vi "Write to File.vi"(8 "error in":errorcluster, 10 "File Actor In":refnum<class "File Actor.lvclass">, 11 "Exe Write Main in":refnum<class "Exe Write Main.lvclass">) -> (0 "error out":errorcluster, 2 "File Actor Out":refnum<class "File Actor.lvclass">)   [LabVIEW 2014, in "Controller.lvlib" / "Exe Write Main.lvclass"]
doc: "In this command, we pole the MAP DVR which contains all of the data that is to be written to file...."
uses:
  Exe Write Main.lvclass
  File Actor/File Actor.lvclass
  File Actor/File Actor.lvclass/File Actor.ctl
  SuperActor/Ex Nested.lvclass/Ex Nested.ctl
  Exe Write Main.lvclass/Exe Write Main.ctl
  reusable/Data/Data.lvclass
  File Actor/Read Save DVR.vi
  File Actor/Read File DVR.vi
  SuperActor/Read Log Session.vi
  <userlib>/_Session Fwk/Session - Root.lvclass
  reusable/Session APIs/Session Log/System Log.lvclass
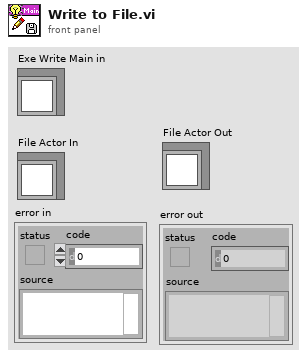
[diagram p1: front panel]
types:
  T1 = typedef "Session - Root.lvclass/Session Handle.ctl" = refnum<data-value>
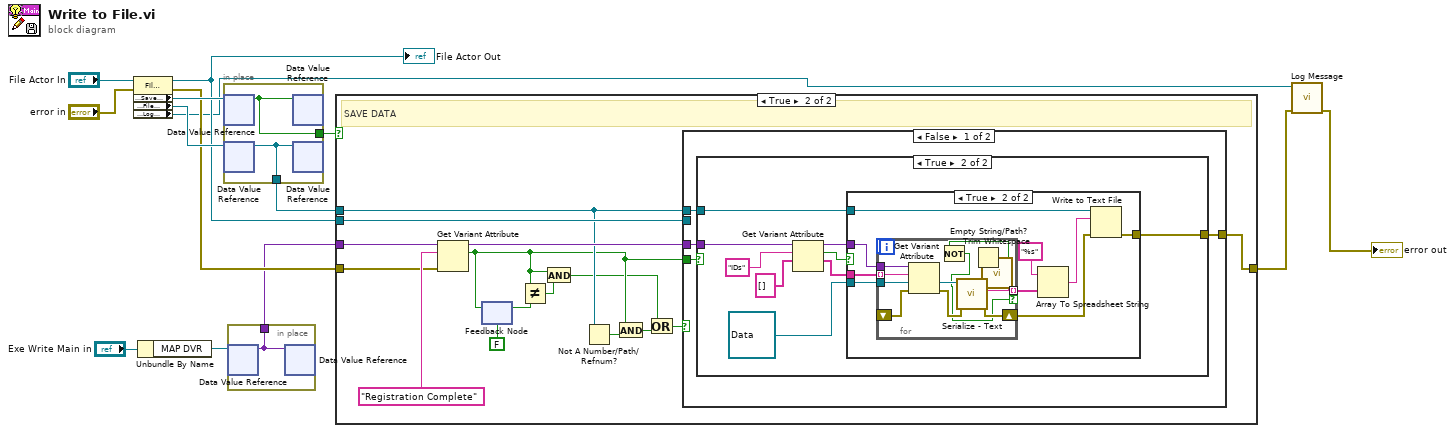
[diagram p0: block diagram]
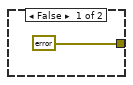
[diagram p4: hidden frame]
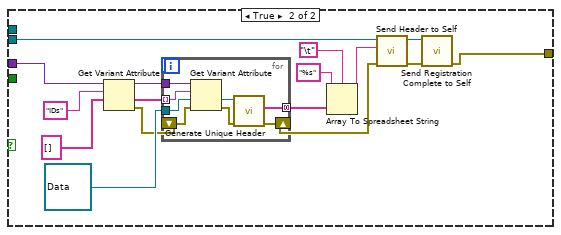
[diagram p5: hidden frame]
diagram:
  n1 = property class="File Actor"(reference="File Actor In", error in="error in") -> (reference out=w4:refnum<class "File Actor.lvclass">, error out=w8:errorcluster, "Accessors:Save DVR"=w13:refnum<data-value>, "Accessors:File DVR"=w11:refnum<data-value>, "Accessors:Log Session"=w3:T1)
  "File Actor Out" <- w4
  n2 = Unbundle By Name("Exe Write Main in") -> ("MAP DVR"=w6:refnum<data-value>)
  n3 = in-place {
    in-place-border: [w16] -> w12
    in-place-border: [w15] -> w10
    n4 = in-place-dvr #1(w13) -> (w16:bool)  [unwired: 1 out]
    n5 = in-place-dvr #2(w11) -> (w15:refnum<file>)  [unwired: 1 out]
    n6 = in-place-dvr #1(w16) -> ()  [unwired: 2 out]
    n7 = in-place-dvr #2(w15) -> ()  [unwired: 2 out]
  }
  n8 = in-place {
    in-place-border: [w17] -> w5
    n9 = in-place-dvr #3(w6) -> (w17:variant)  [unwired: 1 out]
    n10 = in-place-dvr #3(w17) -> ()  [unwired: 2 out]
  }
  n11 = case shown="True" w12 {
    tunnel: [w18 w33] -> w2
    tunnel: w10 -> [_ w24]
    tunnel: w8 -> [w18 w25]
    tunnel: w5 -> [_ w32]
    tunnel: w4 -> [_ w27]
    frame False {
      # "NO SAVE"
    }
    frame True {
      # "SAVE DATA"
      n12 = Get Variant Attribute(Variant=w32, name="Registration Complete", error in=w25) -> (duplicate Variant=w30:variant, found=w22:bool)  [unwired: 1 in, 2 out]
      n13 = feedback-in #4(w22) -> ()
      n14 = feedback #4(FALSE) -> (w29:bool)
      n15 = Not Equal?(x=w22, y=w29) -> (x != y?=w28:bool)
      n16 = And(x=w22, y=w28) -> (x .and. y?=w20:bool)
      n17 = Not A Number/Path/Refnum?(number/path/refnum=w24) -> (NaN/Path/Refnum?=w23:bool)
      n18 = And(x=w22, y=w23) -> (x .and. y?=w21:bool)
      n19 = Or(x=w20, y=w21) -> (x .or. y?=w19:bool)
      n20 = case shown="False" w19 {
        tunnel: [w37 w83] -> w33
        tunnel: w24 -> [w36 _]
        tunnel: w30 -> [w35 w82]
        tunnel: w22 -> [w34 _]
        tunnel: w27 -> [_ w73]
        frame False {
          n21 = case shown="True" w34 {
            tunnel: [_ w46] -> w37
            tunnel: w36 -> [_ w44]
            tunnel: w35 -> [_ w45]
            frame False {
            }
            frame True {
              n22 = Get Variant Attribute(Variant=w45, name="IDs", default value (empty Variant)=string[] []) -> (duplicate Variant=w39:variant, found=w40:bool, value=w41:string[])  [unwired: 1 in, 1 out]
              n23 = case shown="True" w40 {
                tunnel: w41 -> [_ w56]
                tunnel: w39 -> [_ w55]
                tunnel: refnum<class "Data.lvclass"> refnum ("Base Data Lib:Data") -> [_ w54]
                tunnel: w44 -> [_ w50]
                tunnel: [errorcluster {"status"=FALSE, "code"=0, "source"=""} ("error out") w49] -> w46
                frame False {
                }
                frame True {
                  n24 = for {
                    tunnel: w56 -> [w66] mode=indexing
                    tunnel: w55 -> [w67]
                    tunnel: w54 -> [w65]
                    tunnel: [w57] -> w53 mode=indexing if=w59
                    shift-right: [w62] -> w48
                    shift-left: _ -> [w61]
                    n25 = Get Variant Attribute(Variant=w67, name=w66, default value (empty Variant)=w65, error in=w61) -> (value=w64:refnum<class "Data.lvclass">, error out=w63:errorcluster)  [unwired: 2 out]
                    n26 = call-dynamic "Serialize - Text.vi"("error in"=w63, "Data in"=w64) -> ("error out"=w62:errorcluster, "Serialized Text"=w58:string)  [unwired: 7 in, 1 out]
                    n27 = Empty String/Path?(string/path=w58) -> (empty?=w60:bool)
                    n28 = Not(x=w60) -> (.not. x?=w59:bool)
                    n29 = call <vilib>:"Trim Whitespace.vi"("string"=w58) -> ("trimmed string"=w57:string)  [unwired: 1 in]
                  }
                  n30 = Array To Spreadsheet String(array=w53, 3:"%s" ("format string")) -> (spreadsheet string=w51:string)  [unwired: 1 in]
                  n31 = Write to Text File(file (use dialog)=w50, text=w51, error in=w48) -> (error out=w49:errorcluster)  [unwired: 1 in, 2 out]
                }
              }
            }
          }
        }
        frame True {
          n32 = Get Variant Attribute(Variant=w82, name="IDs", default value (empty Variant)=string[] []) -> (duplicate Variant=w78:variant, value=w79:string[], error out=w69:errorcluster)  [unwired: 1 in, 1 out]
          n33 = for {
            tunnel: w79 -> [w91] mode=indexing
            tunnel: w78 -> [w90]
            tunnel: refnum<class "Data.lvclass"> refnum ("Base Data Lib:Data") -> [w89]
            tunnel: [w87] -> w76 mode=concatenating
            shift-right: [w84] -> w68
            shift-left: w69 -> [w85]
            n34 = Get Variant Attribute(Variant=w90, name=w91, default value (empty Variant)=w89, error in=w85) -> (value=w88:refnum<class "Data.lvclass">, error out=w86:errorcluster)  [unwired: 2 out]
            n35 = call-dynamic "Generate Unique Header.vi"("error in"=w86, "Data in"=w88) -> ("error out"=w84:errorcluster, "Header"=w87:string[])  [unwired: 7 in, 1 out]
          }
          n36 = Array To Spreadsheet String(delimiter (Tab)="\t", array=w76, 3:"%s" ("format string")) -> (spreadsheet string=w71:string)
          n37 = call "Send Header to Self.vi"("error in"=w68, "Header"=w71, "File Actor in"=w73) -> ("error out"=w70:errorcluster, "File Actor out"=w72:refnum<class "File Actor.lvclass">)  [unwired: 7 in]
          n38 = call "Send Registration Complete to Self.vi"("error in (no error)"=w70, "File Actor in"=w72) -> ("error out"=w83:errorcluster)  [unwired: 8 in, 1 out]
        }
      }
    }
  }
  n39 = call "Log Message.vi"("error in"=w2, "session in"=w3) -> ("error out"=→"error out":errorcluster)  [unwired: 8 in, 1 out]
